vi "Chameleon Send Cmd.vi"(0 "VISA Ref":refnum<visa-resource-name>, 7 "Command":string, 11 "Error In":errorcluster) -> (4 "VISA Ref Out":refnum<visa-resource-name>, 8 "Response":string, 15 "Error Out":errorcluster)   [LabVIEW 2020]
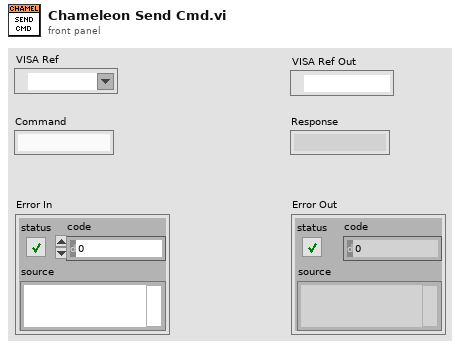
[diagram p1: front panel]
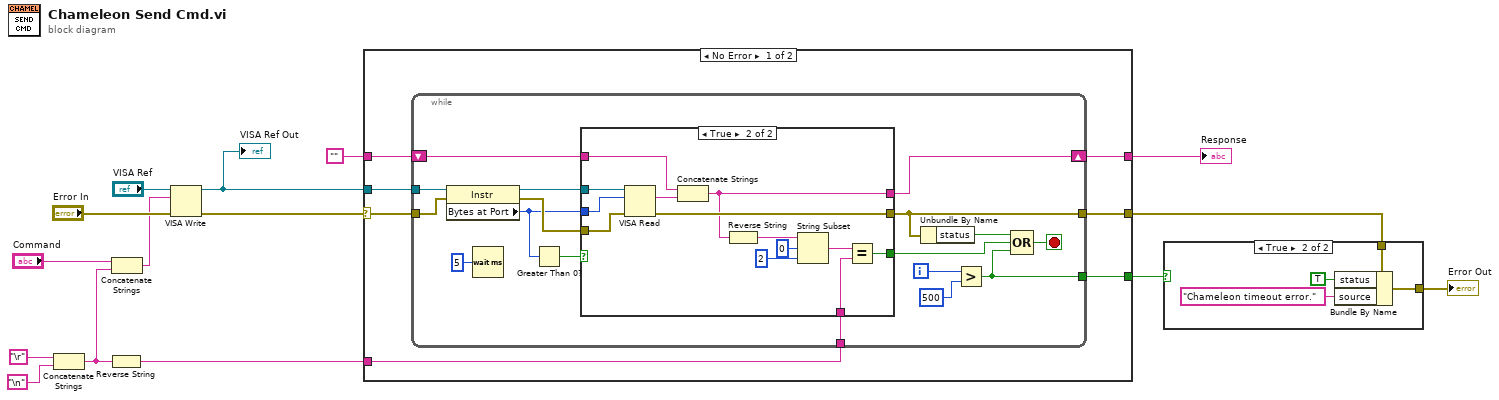
[diagram p0: block diagram]
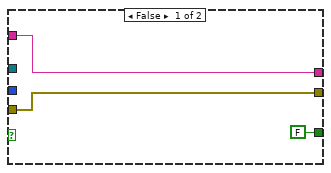
[diagram p3: hidden frame]
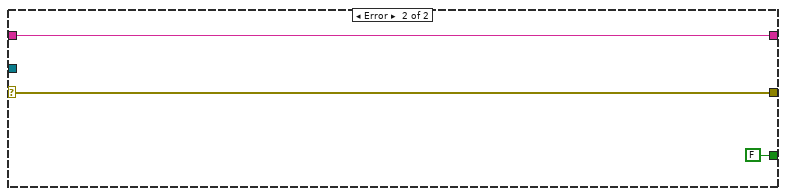
[diagram p4: hidden frame]
diagram:
  n1 = Concatenate Strings("\r", "\n") -> (w6:string)
  n2 = Reverse String(1:w6) -> (0:w5:string)
  n3 = Concatenate Strings("Command", w6) -> (w9:string)
  n4 = VISA Write(VISA resource name="VISA Ref", write buffer=w9, error in (no error)="Error In") -> (VISA resource name out=w10:refnum<visa-resource-name>, error out=w11:errorcluster)  [unwired: 1 out]
  "VISA Ref Out" <- w10
  n5 = case shown="No Error" w11 {
    selector: w11 -> [w16 w57]
    tunnel: w10 -> [w17 _]
    tunnel: "" -> [w22 w58]
    tunnel: [w21 w58] -> w4
    tunnel: [w20 w57] -> w2
    tunnel: [w19 FALSE] -> w3
    tunnel: w5 -> [w18 _]
    frame No Error {
      n6 = while {
        tunnel: w17 -> [w39]
        tunnel: w16 -> [w38]
        shift-right: [w28] -> w21
        shift-left: w22 -> [w29]
        tunnel: [w25] -> w20
        tunnel: [w24] -> w19
        tunnel: w18 -> [w23]
        i -> [w37]
        stop <- w35 stop-if-true
        n7 = property class="Instr"(reference=w39, error in=w38) -> (reference out=w31:refnum<visa-resource-name>, error out=w32:errorcluster, "Bytes at Port"=w30:u32)
        n8 = Wait (ms)(milliseconds to wait=u32 5) -> ()  [unwired: 1 out]
        n9 = Greater Than 0?(x=w30) -> (x > 0?=w33:bool)
        n10 = case shown="True" w33 {
          tunnel: w32 -> [w41 w54]
          tunnel: w31 -> [_ w55]
          tunnel: w30 -> [_ w53]
          tunnel: w29 -> [w42 w52]
          tunnel: [w42 w49] -> w28
          tunnel: [w41 w50] -> w25
          tunnel: [FALSE w44] -> w26
          tunnel: w23 -> [_ w43]
          frame False {
          }
          frame True {
            n11 = VISA Read(VISA resource name=w55, byte count=w53, error in (no error)=w54) -> (read buffer=w51:string, error out=w50:errorcluster)  [unwired: 2 out]
            n12 = Concatenate Strings(w52, w51) -> (w49:string)
            n13 = Reverse String(1:w49) -> (0:w48:string)
            n14 = String Subset(string=w48, offset (0)=0, length (rest)=2 ("length (rest)")) -> (substring=w45:string)
            n15 = Equal?(x=w45, y=w43) -> (x = y?=w44:bool)
          }
        }
        n16 = Unbundle By Name(w25) -> ("status"=w27:bool)
        n17 = Greater?(x=w37, y=500) -> (0:w24:bool)
        n18 = Compound Arithmetic op=OR(w27, w26, w24) -> (w35:bool)
      }
    }
    frame Error {
    }
  }
  "Response" <- w4
  n19 = case shown="True" w3 {
    tunnel: w2 -> [w59 w63]
    tunnel: [w59 w60] -> w1
    frame False {
    }
    frame True {
      n20 = Bundle By Name(cluster=w63, "status"=TRUE, "source"="Chameleon timeout error.") -> (w60:errorcluster)
    }
  }
  "Error Out" <- w1
